vi "TimedFacade.vi"(0 "Data In":T4, 2 "Display State In":T2, 3 "Container State":T3) -> (6 "Data Out":T4, 7 "Display State Out":T2, 8 "Action":T1)   [LabVIEW 2018, in "Ui.lvlib" / "Timed.xctl"]
uses:
  Timed.xctl
  TimedData.ctl
  <vilib>/_xctls/Container State.ctl
  TimedState.ctl
  <vilib>/_xctls/Action.ctl
  <vilib>/_xctls/XControlSupport.lvlib
panel:
  in  "Frequency":dbl[unit](knob) scale=0.0..100.0
  in  "Start":bool
  in  "Stop":bool
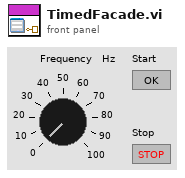
[diagram p1: front panel]
types:
  T1 = typedef "XControlSupport.lvlib/Action.ctl" = cluster{"Data Changed?":bool, "State Changed?":bool, "Action Name":string}
  T2 = typedef "Ui.lvlib/Timed.xctl/TimedState.ctl" = cluster{"Start Visible":bool}
  T3 = typedef "XControlSupport.lvlib/Container State.ctl" = cluster{"Indicator?":bool, "Run Mode?":bool, " Refnum":refnum<vi>}
  T4 = typedef "Ui.lvlib/Timed.xctl/TimedData.ctl" = cluster{"Stop":bool, "Start":bool, "Time (ms)":i64}
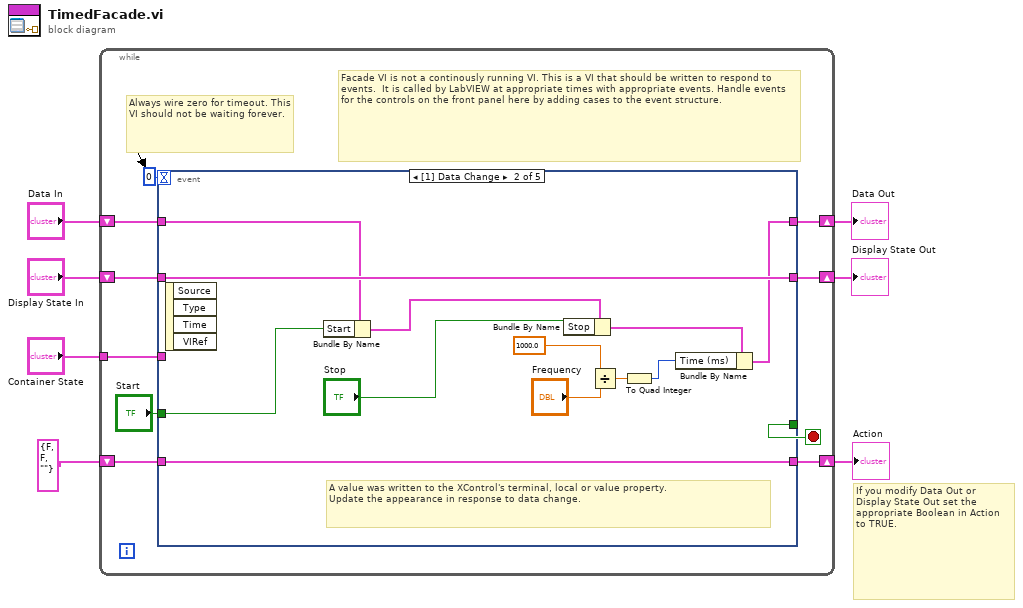
[diagram p0: block diagram]
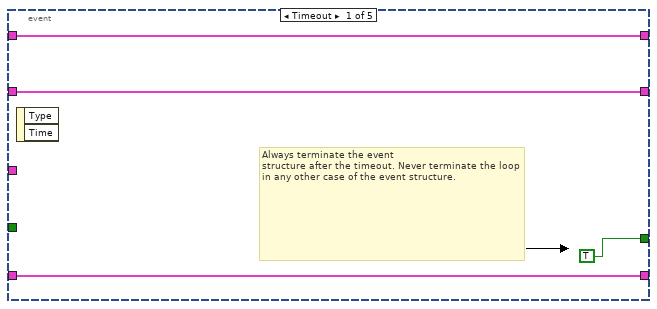
[diagram p2: hidden frame]
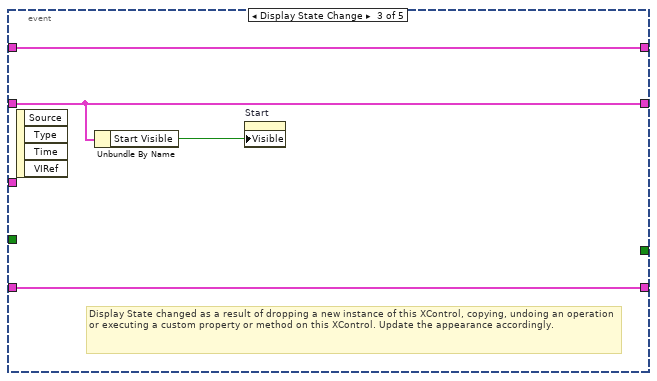
[diagram p3: hidden frame]
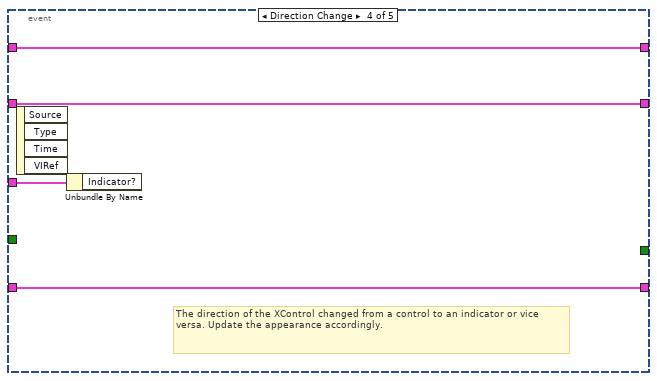
[diagram p4: hidden frame]
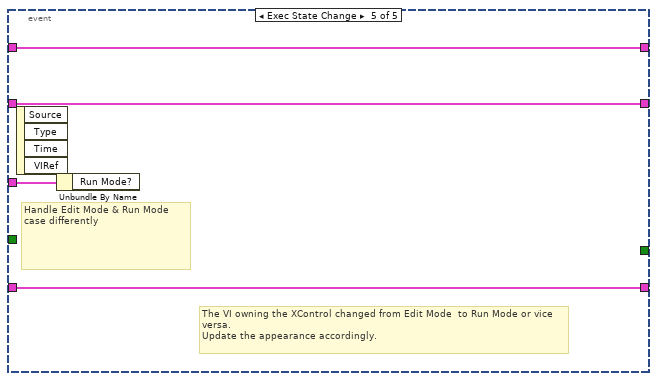
[diagram p5: hidden frame]
diagram:
  # "If you modify Data Out or\nDisplay State Out set the\nappropriate Boolean in Action\nto TRUE."
  n1 = while {
    shift-right: [w16] -> w4
    shift-left: "Display State In" -> [w17]
    tunnel: "Container State" -> [w13]
    shift-right: [w11] -> w7
    shift-left: "Data In" -> [w12]
    shift-right: [w9] -> w2
    shift-left: T1 {"Data Changed?"=FALSE, "State Changed?"=FALSE, "Action Name"=""} ("Action") -> [w10]
    stop <- w15 stop-if-true
    # "Facade VI is not a continously running VI. This is a VI that should be written to respond to events.  It is called by LabVIEW at appropriate times with appropriate events. Handle events for the controls on the front panel here by adding cases to the event structure."
    # "Always wire zero for timeout. This\nVI should not be waiting forever."
    n2 = event shown="[1] Data Change" {
      selector: _ -> [_ _ _ _ _]
      dyn-events: _ -> [_ _ _ _ _]
      timeout: 0 -> [_ _ _ _ _]
      tunnel: w17 -> [w19 w33 w35 w40 w44]
      tunnel: [w19 w33 w35 w40 w44] -> w16
      tunnel: [TRUE _ _ _ _] -> w15
      tunnel: w13 -> [_ _ _ w41 w45]
      tunnel: w12 -> [w18 w30 w37 w39 w43]
      tunnel: [w18 w23 w37 w39 w43] -> w11
      tunnel: [w20 w22 w36 w38 w42] -> w9
      tunnel: w10 -> [w20 w22 w36 w38 w42]
      tunnel: "Start" -> [_ w31 _ _ _]
      event Timeout {
        # "Always terminate the event\nstructure after the timeout. Never terminate the loop in any other case of the event structure."
        n3 = event-data() -> ()  [unwired: 1 in, 2 out]
      }
      event Data Change {
        # "A value was written to the XControl's terminal, local or value property.\nUpdate the appearance in response to data change."
        n4 = event-data() -> ()  [unwired: 1 in, 4 out]
        n5 = Bundle By Name(cluster=w30, "Start"=w31) -> (w32:T4)
        n6 = Bundle By Name(cluster=w32, "Stop"="Stop") -> (w24:T4)
        n7 = Divide(x=dbl[unit] 1000.0, y="Frequency") -> (x/y=w26:dbl)
        n8 = To Quad Integer(1:w26) -> (0:w25:i64)
        n9 = Bundle By Name(cluster=w24, "Time (ms)"=w25) -> (w23:T4)
      }
      event Display State Change {
        # "Display State changed as a result of dropping a new instance of this XControl, copying, undoing an operation or executing a custom property or method on this XControl. Update the appearance accordingly."
        n10 = event-data() -> ()  [unwired: 1 in, 4 out]
        n11 = Unbundle By Name(w35) -> ("Start Visible"=w34:bool)
        n12 = property on="Start" class="Bool"("Visible"=w34) -> ()  [unwired: 2 in, 2 out]
      }
      event Direction Change {
        # "The direction of the XControl changed from a control to an indicator or vice versa. Update the appearance accordingly."
        n13 = event-data() -> ()  [unwired: 1 in, 4 out]
        n14 = Unbundle By Name(w41) -> ()  [unwired: 1 out]
      }
      event Exec State Change {
        # "The VI owning the XControl changed from Edit Mode  to Run Mode or vice versa.\nUpdate the appearance accordingly."
        # "Handle Edit Mode & Run Mode\ncase differently"
        n15 = event-data() -> ()  [unwired: 1 in, 4 out]
        n16 = Unbundle By Name(w45) -> ()  [unwired: 1 out]
      }
    }
  }
  "Display State Out" <- w4
  "Data Out" <- w7
  "Action" <- w2
